vi "Day02-01_연습문제.vi"() -> ()   [LabVIEW 2021]
panel:
  out "배열 2":i32[][](array[numeric])
  out "숫자별 횟수":dbl[](array[numeric])
  out "주사위 던진 횟수":i32
  out "랜덤 주사위 값":dbl[](array[numeric])
  out "배열":i32[][](array[numeric])
  # "p.198 문제 1-3. 구구단 출력 (2중 for 문 사용)"
  # "p.197 문제 1-2. 랜덤 주사위(0~6)를 20개 발생시키고 각 숫자가 발생한 개수 카운트"
  # "0"
  # "1"
  # "2"
  # "3"
  # "4"
  # "5"
  # "6"
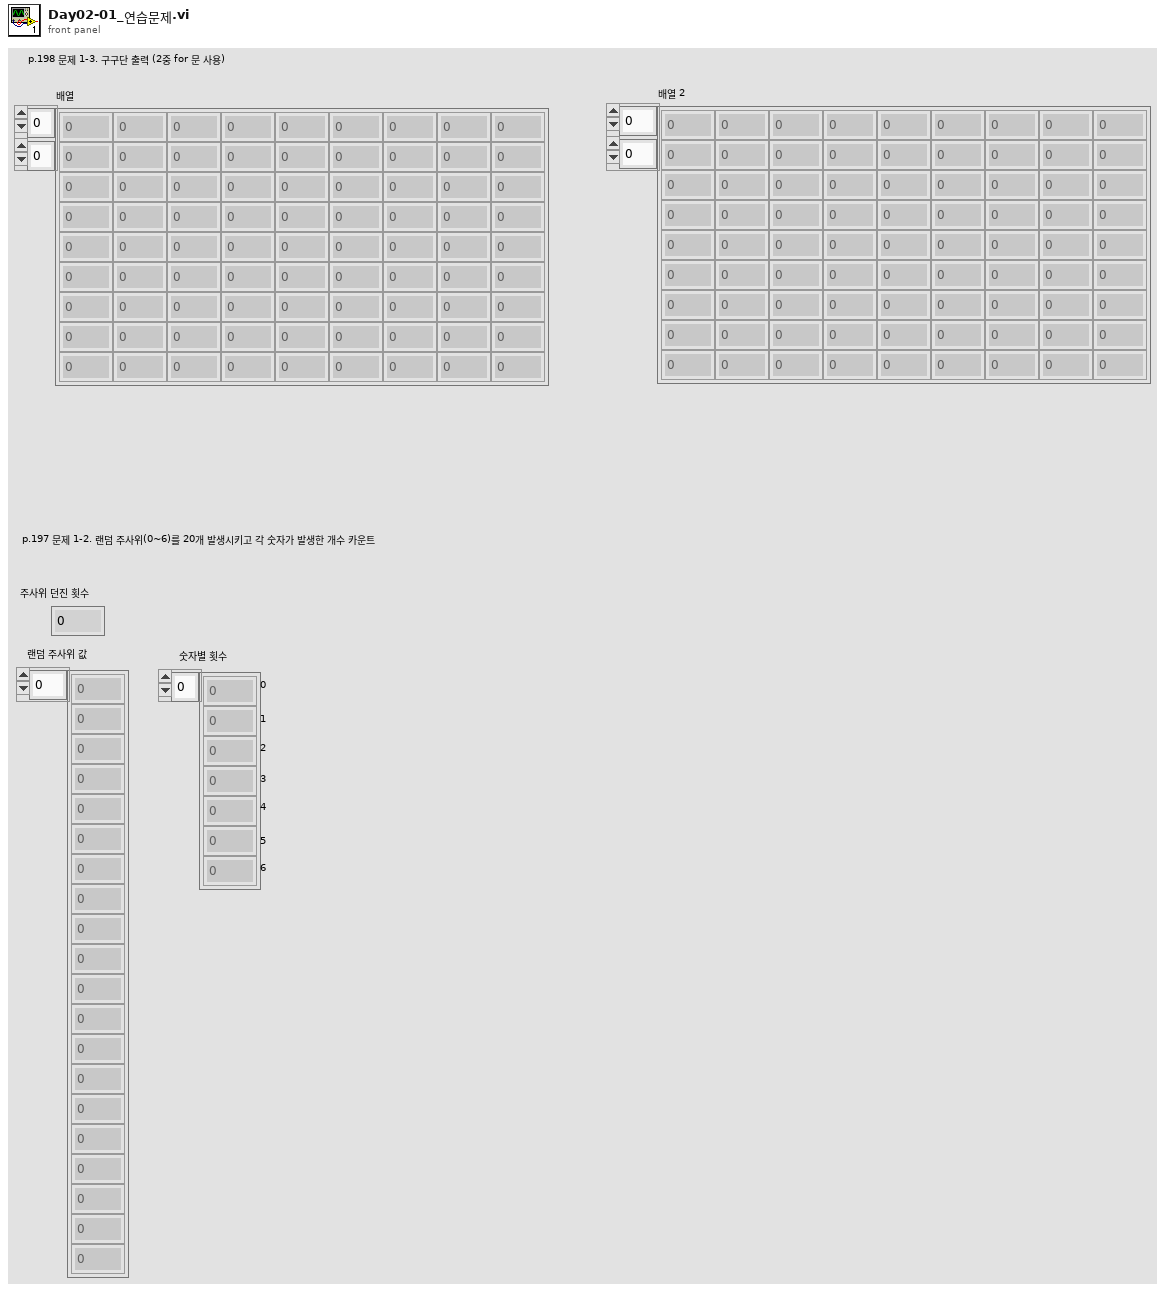
[diagram p1: front panel]
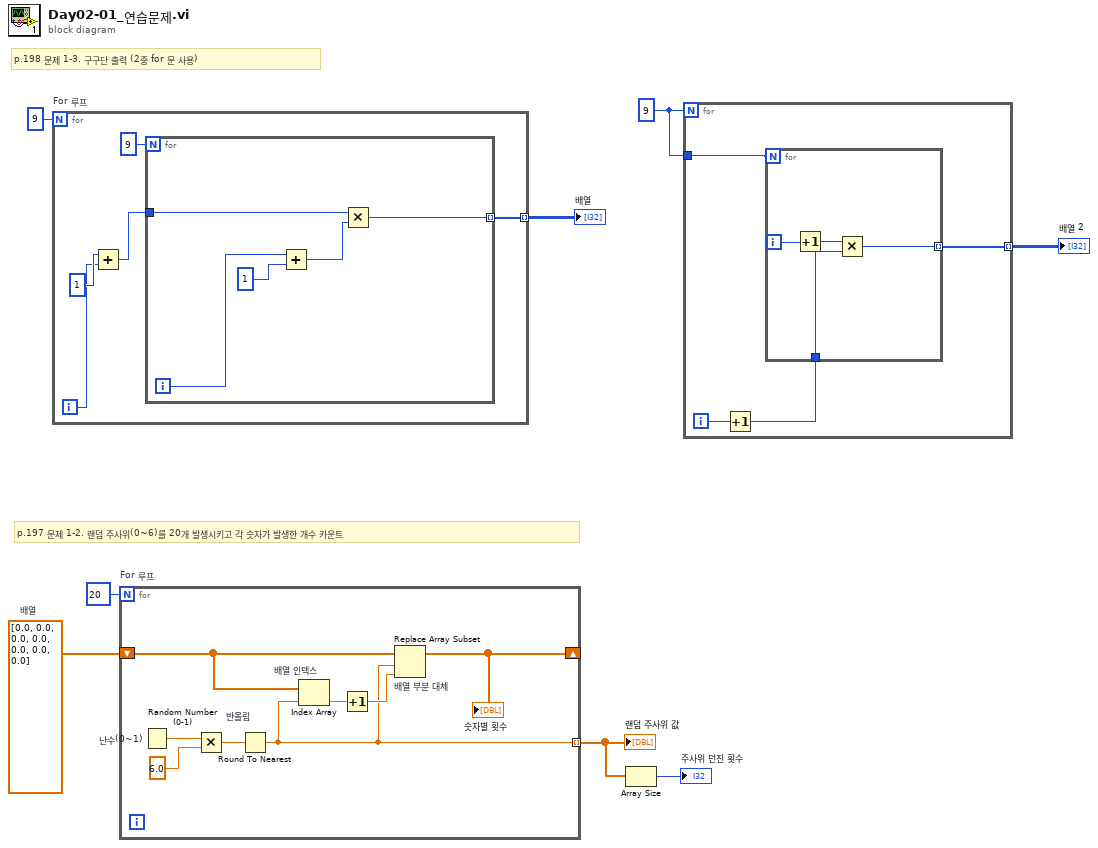
[diagram p0: block diagram]
diagram:
  w2 = 9
  w3 = dbl[] [0.0, 0.0, 0.0, 0.0, 0.0, 0.0, 0.0]  # 배열
  # "p.197 문제 1-2. 랜덤 주사위(0~6)를 20개 발생시키고 각 숫자가 발생한 개수 카운트"
  # "p.198 문제 1-3. 구구단 출력 (2중 for 문 사용)"
  n1 = for "For 루프" {
    N: 9 -> [_]
    tunnel: [w9] -> w7 mode=indexing
    i -> [w11]
    n2 = Add(x=1 ("y"), y=w11) -> (x+y=w10:i32)
    n3 = for {
      N: 9 -> [_]
      tunnel: w10 -> [w16]
      tunnel: [w14] -> w9 mode=indexing
      i -> [w18]
      n4 = Add(x=w18, y=1) -> (x+y=w15:i32)
      n5 = Multiply(x=w16, y=w15) -> (x*y=w14:i32)
    }
  }
  "배열" <- w7
  n6 = for "For 루프" {
    N: 20 -> [_]
    tunnel: [w20] -> w5 mode=indexing
    shift-right: [w23] -> _
    shift-left: w3 -> [w21]
    n7 = Random Number (0-1) "난수(0~1)"() -> (number: 0 to 1=w26:dbl)
    n8 = Multiply(x=w26, y=6.0) -> (x*y=w24:dbl)
    n9 = Round To Nearest "반올림"(number=w24) -> (nearest integer value=w20:dbl)
    n10 = Index Array "배열 인덱스"(array=w21, index=w20) -> (element=w19:dbl)
    n11 = Increment(x=w19) -> (x+1=w22:dbl)
    n12 = Replace Array Subset "배열 부분 대체"(array=w21, new element=w22, index=w20) -> (w23:dbl[])
    "숫자별 횟수" <- w23
  }
  "랜덤 주사위 값" <- w5
  n13 = Array Size(array=w5) -> (size(s)=→"주사위 던진 횟수":i32)
  n14 = for {
    N: w2 -> [_]
    tunnel: w2 -> [w30]
    tunnel: [w27] -> w1 mode=indexing
    i -> [w29]
    n15 = Increment(x=w29) -> (x+1=w28:i32)
    n16 = for {
      N: w30 -> [_]
      tunnel: w28 -> [w32]
      tunnel: [w31] -> w27 mode=indexing
      i -> [w33]
      n17 = Increment(x=w33) -> (x+1=w34:i32)
      n18 = Multiply(x=w34, y=w32) -> (x*y=w31:i32)
    }
  }
  "배열 2" <- w1
